vi "Read.Pcap.File.vi"(8 "error in":errorcluster, 11 "Path":path=path "F:/work/fpganow/Market.Data.PoC/submodules/cboe_pitch/generated_2025_02_09.pcap") -> (0 "error out":errorcluster={"status"=TRUE, "code"=7, "source"="Open/Create/Replace File in Read.Pcap.File.vi<APPEND>\nc:\\work\\git\\fpganow\\Market.Data.PoC\\submodules\\cboe_pitch\\generated_2025_02_09.pcap"}, 1 "Records":T1[](array[typedef]) {"ts_sec" format="%.0x"; "ts_usec" format="%.0x"; "incl_len" format="%.0x"; "orig_len" format="%.0x"; "payload" format="%.0x"}, 2 "Global\nHeader":T2={"magic_number"=3569595041, "version_major"=512, "version_minor"=1024, "thiszone"=0, "sigfigs"=0, "snap_len"=1024, "network"=16777216} {"magic_number" format="%.0x"; "version_major" format="%.0x"; "version_minor" format="%.0x"; "thiszone" format="%.0x"; "sigfigs" format="%.0x"; "network" format="%.0x"}, 3 "Swap?":bool)   [LabVIEW 2020]
uses:
  Global.Header.ctl
  record.ctl
panel:
  out "path out":path=path "F:/work/fpganow/Market.Data.PoC"
  out "# of Records":i32
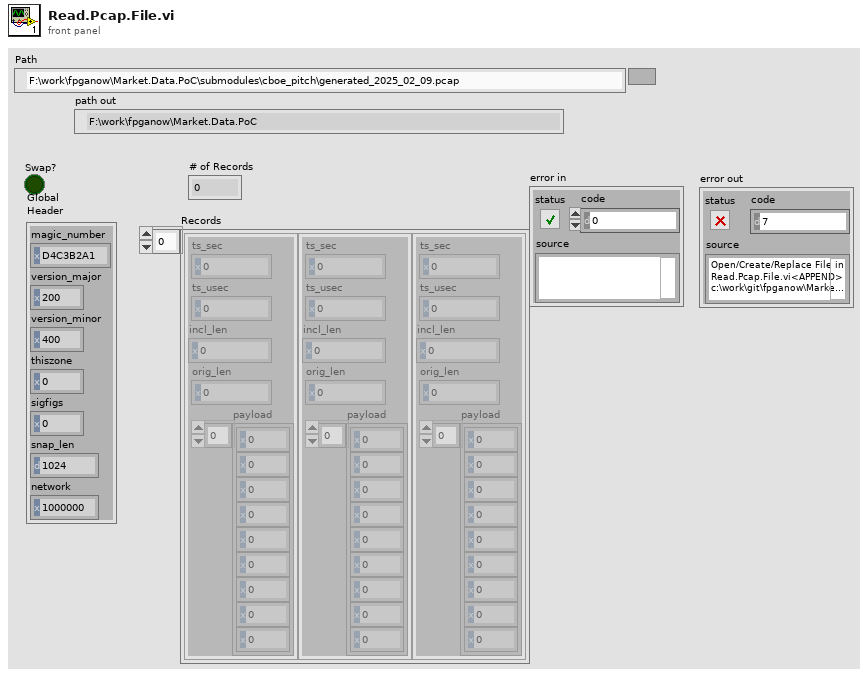
[diagram p1: front panel]
types:
  T1 = typedef "record.ctl" = cluster{"ts_sec":u32, "ts_usec":u32, "incl_len":u32, "orig_len":u32, "payload":u8[]}
  T2 = typedef "global.header.ctl" = cluster{"magic_number":u32, "version_major":u16, "version_minor":u16, "thiszone":u32, "sigfigs":u32, "snap_len":u32, "network":u32}
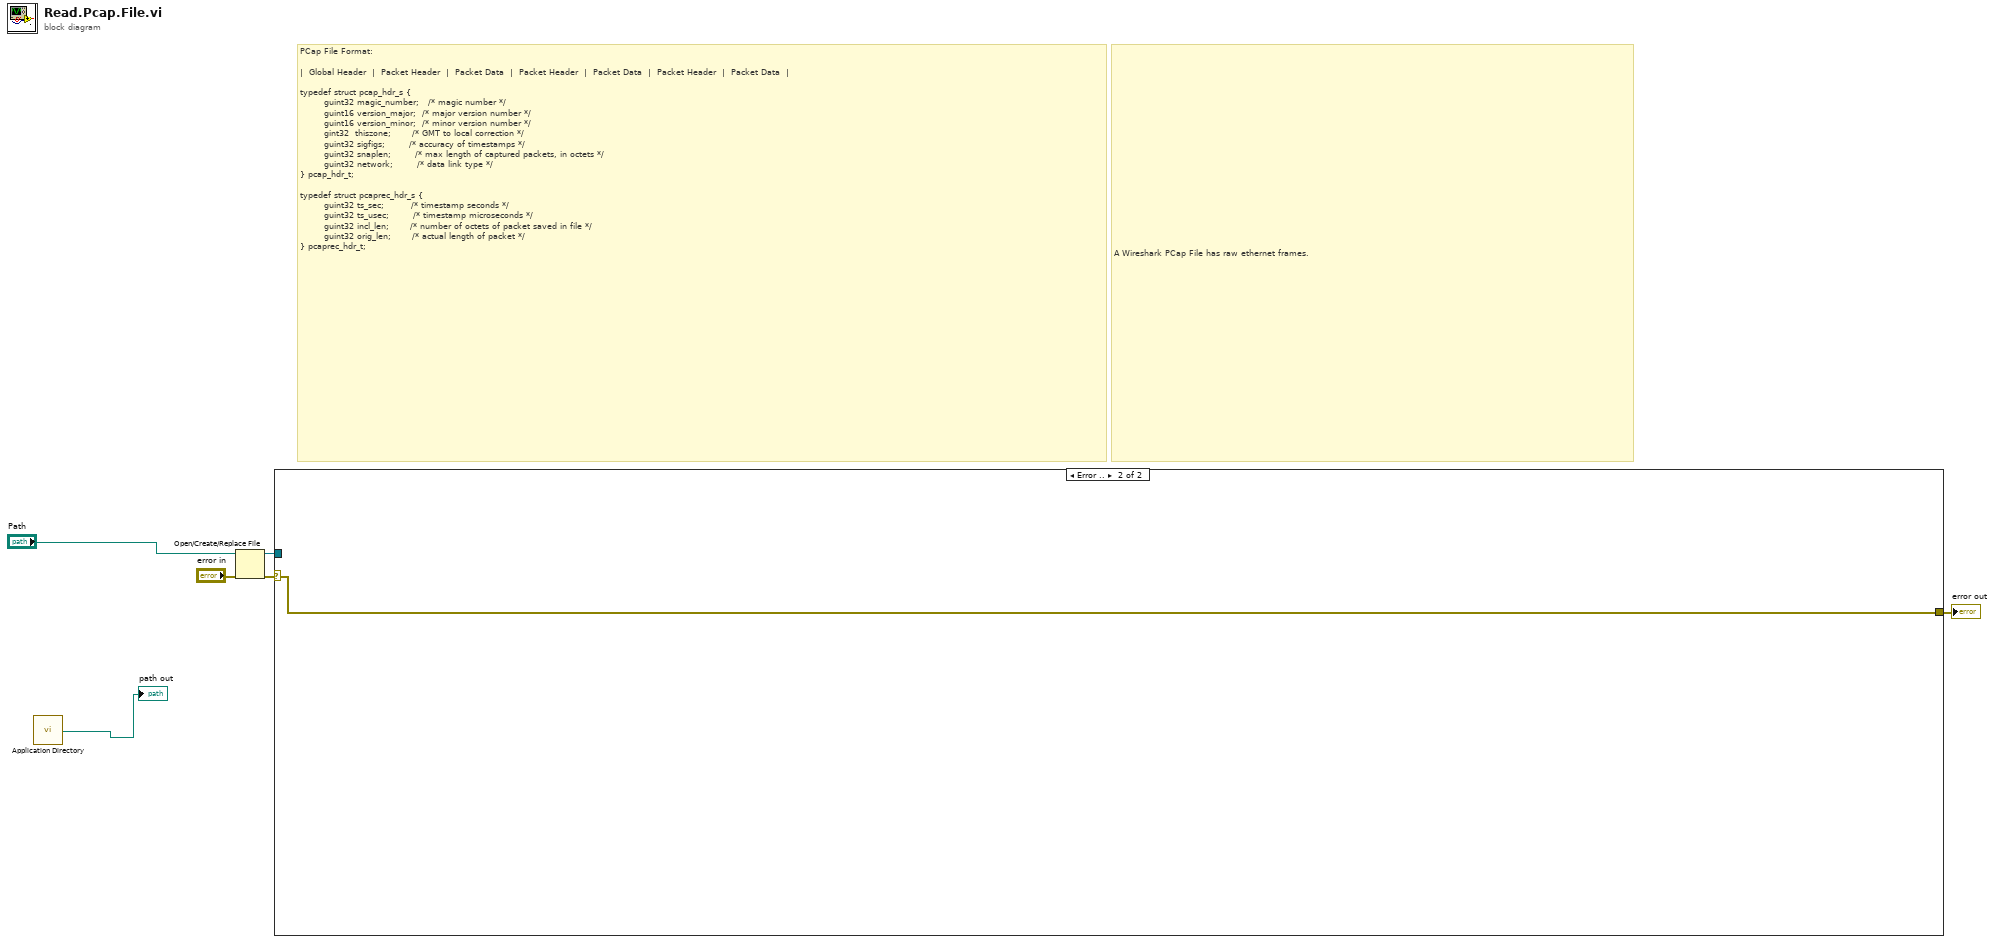
[diagram p0: block diagram]
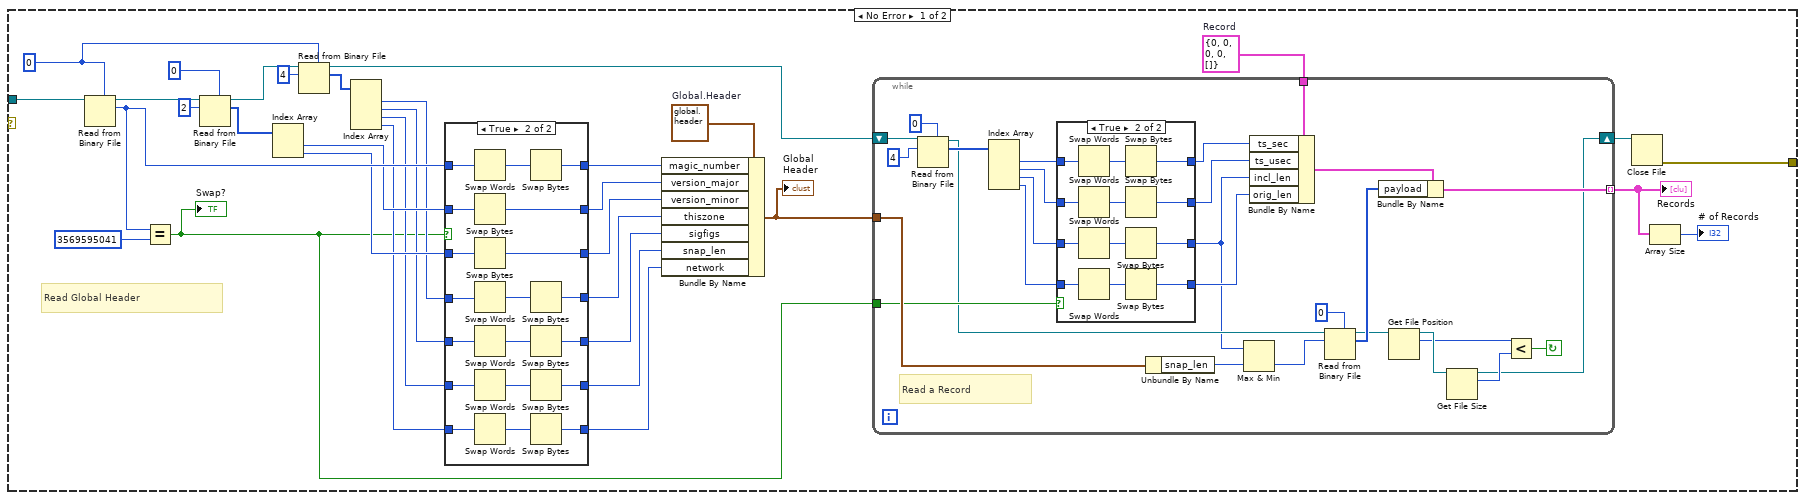
[diagram p2: hidden frame]
diagram:
  # "A Wireshark PCap File has raw ethernet frames."
  # "PCap File Format:\n\n|  Global Header  |  Packet Header  |  Packet Data  |  Packet Header  |  Packet Data  |  Packet Header  |  Packet Data  |\n\ntypedef struct pcap_hdr_s {\n        guint32 magic_number;   /* magic number */\n        guint16 version_major;  /* major version number */\n        guint16 version_minor;  /* minor version number */\n        gint32  thiszone;       /* GMT to local correction */\n        guint32 sigfigs;        /* accuracy of timestamps */\n        guint32 snaplen;        /* max length of captured packets, in octets */\n        guint32 network;        /* data link type */\n} pcap_hdr_t;\n\ntypedef struct pcaprec_hdr_s {\n        guint32 ts_sec;         /* timestamp seconds */\n        guint32 ts_usec;        /* timestamp microseconds */\n        guint32 incl_len;       /* number of octets of packet saved in file */\n        guint32 orig_len;       /* actual length of packet */\n} pcaprec_hdr_t;"
  n1 = call <vilib>:"Application Directory.vi"() -> ("Application Directory"=→"path out":path)
  n2 = Open/Create/Replace File(file path (use dialog)="Path", error in="error in") -> (refnum out=w4:refnum<file>, error out=w5:errorcluster)  [unwired: 4 in, 1 out]
  n3 = case shown="Error .." w5 {
    selector: w5 -> [_ w110]
    tunnel: w4 -> [w39 _]
    tunnel: [w7 w110] -> w3
    frame No Error {
      w8 = T1 {"ts_sec"=0, "ts_usec"=0, "incl_len"=0, "orig_len"=0, "payload"=[]}  # Record
      w9 = T2 {"magic_number"=3569595041, "version_major"=512, "version_minor"=1024, "thiszone"=0, "sigfigs"=0, "snap_len"=1024, "network"=16777216}  # Global.Header
      w32 = u32 0
      # "Read Global Header"
      n4 = Read from Binary File(5:w32, 11:w39) -> (2:w29:u32, 3:w36:refnum<file>)  [unwired: 4 in, 2 out]
      n5 = Equal?(x=w29, y=u32 3569595041) -> (x = y?=w11:bool)
      "Swap?" <- w11
      n6 = Read from Binary File(5:u16 0, 10:2 ("count (1)"), 11:w36) -> (2:w34:u16[], 3:w33:refnum<file>)  [unwired: 3 in, 2 out]
      n7 = Index Array(array=w34) -> (element #1=w27:u16, element #2=w26:u16)  [unwired: 2 in]
      n8 = Read from Binary File(5:w32, 10:4 ("count (1)"), 11:w33) -> (2:w30:u32[], 3:w15:refnum<file>)  [unwired: 3 in, 2 out]
      n9 = Index Array(array=w30) -> (element #1=w23:u32, element #2=w21:u32, element #3=w20:u32, element #4=w19:u32)  [unwired: 4 in]
      n10 = case shown="True" w11 {
        tunnel: w29 -> [w90 w109]
        tunnel: [w90 w107] -> w28
        tunnel: w27 -> [w89 w106]
        tunnel: w26 -> [w88 w105]
        tunnel: [w89 w104] -> w25
        tunnel: [w88 w103] -> w24
        tunnel: w23 -> [w87 w98]
        tunnel: [w87 w97] -> w22
        tunnel: w21 -> [w86 w96]
        tunnel: w20 -> [w85 w95]
        tunnel: w19 -> [w84 w94]
        tunnel: [w86 w93] -> w18
        tunnel: [w85 w92] -> w17
        tunnel: [w84 w91] -> w16
        frame False {
        }
        frame True {
          n11 = Swap Words(1:w109) -> (0:w108:u32)
          n12 = Swap Bytes(anything=w106) -> (byte swapped=w104:u16)
          n13 = Swap Bytes(anything=w105) -> (byte swapped=w103:u16)
          n14 = Swap Words(1:w98) -> (0:w102:u32)
          n15 = Swap Words(1:w96) -> (0:w101:u32)
          n16 = Swap Words(1:w95) -> (0:w100:u32)
          n17 = Swap Words(1:w94) -> (0:w99:u32)
          n18 = Swap Bytes(anything=w108) -> (byte swapped=w107:u32)
          n19 = Swap Bytes(anything=w102) -> (byte swapped=w97:u32)
          n20 = Swap Bytes(anything=w101) -> (byte swapped=w93:u32)
          n21 = Swap Bytes(anything=w100) -> (byte swapped=w92:u32)
          n22 = Swap Bytes(anything=w99) -> (byte swapped=w91:u32)
        }
      }
      n23 = Bundle By Name(cluster=w9, "magic_number"=w28, "version_major"=w25, "version_minor"=w24, "thiszone"=w22, "sigfigs"=w18, "snap_len"=w17, "network"=w16) -> (w10:T2)
      "Global\nHeader" <- w10
      n24 = while {
        tunnel: w8 -> [w63]
        tunnel: [w54] -> w13 mode=indexing
        shift-right: [w53] -> w14
        shift-left: w15 -> [w67]
        tunnel: w10 -> [w51]
        tunnel: w11 -> [w49]
        stop <- w55 continue-if-true
        # "Read a Record"
        n25 = Read from Binary File(5:u32 0 ("count (1)"), 10:4 ("count (1)"), 11:w67) -> (2:w64:u32[], 3:w46:refnum<file>)  [unwired: 3 in, 2 out]
        n26 = Index Array(array=w64) -> (element #1=w48:u32, element #2=w45:u32, element #3=w44:u32, element #4=w43:u32)  [unwired: 4 in]
        n27 = case shown="True" w49 {
          tunnel: w48 -> [w71 w83]
          tunnel: [w71 w81] -> w47
          tunnel: w45 -> [w70 w80]
          tunnel: w44 -> [w69 w78]
          tunnel: w43 -> [w68 w77]
          tunnel: [w70 w74] -> w42
          tunnel: [w69 w73] -> w40
          tunnel: [w68 w72] -> w41
          frame False {
          }
          frame True {
            n28 = Swap Words(1:w83) -> (0:w82:u32)
            n29 = Swap Words(1:w80) -> (0:w79:u32)
            n30 = Swap Words(1:w78) -> (0:w75:u32)
            n31 = Swap Words(1:w77) -> (0:w76:u32)
            n32 = Swap Bytes(anything=w82) -> (byte swapped=w81:u32)
            n33 = Swap Bytes(anything=w79) -> (byte swapped=w74:u32)
            n34 = Swap Bytes(anything=w75) -> (byte swapped=w73:u32)
            n35 = Swap Bytes(anything=w76) -> (byte swapped=w72:u32)
          }
        }
        n36 = Unbundle By Name(w51) -> ("snap_len"=w50:u32)
        n37 = Max & Min(x=w40, y=w50) -> (min(x,y)=w52:u32)  [unwired: 1 out]
        n38 = Bundle By Name(cluster=w63, "ts_sec"=w47, "ts_usec"=w42, "incl_len"=w40, "orig_len"=w41) -> (w61:T1)
        n39 = Read from Binary File(5:u8 0 ("count (1)"), 10:w52, 11:w46) -> (2:w60:u8[], 3:w59:refnum<file>)  [unwired: 3 in, 2 out]
        n40 = Bundle By Name(cluster=w61, "payload"=w60) -> (w54:T1)
        n41 = Get File Position(7:w59) -> (2:w57:i64, 3:w58:refnum<file>)  [unwired: 1 in, 1 out]
        n42 = Get File Size(file=w58) -> (refnum out=w53:refnum<file>, size (in bytes)=w56:i64)  [unwired: 1 in, 1 out]
        n43 = Less?(x=w57, y=w56) -> (x < y?=w55:bool)
      }
      "Records" <- w13
      n44 = Close File(refnum=w14) -> (error out=w7:errorcluster)  [unwired: 1 in, 1 out]
      n45 = Array Size(array=w13) -> (size(s)=→"# of Records":i32)
    }
    frame Error {
    }
  }
  "error out" <- w3
